vi "PIDByError.vi"(0 "Error":dbl, 1 "PID Gains":cluster{"P":dbl, "I":dbl, "D":dbl}, 2 "Init":bool, 3 "Reset":bool) -> (7 "Control":dbl)   [LabVIEW 2013, in "ProcessorHelperFunctions.lvlib"]
uses:
  ProcessorHelperFunctions.lvlib
  <vilib>/ptbypt/NI_PtbyPt.lvlib
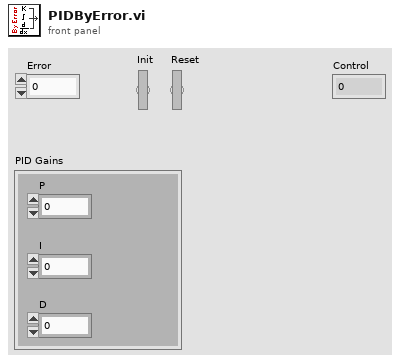
[diagram p1: front panel]
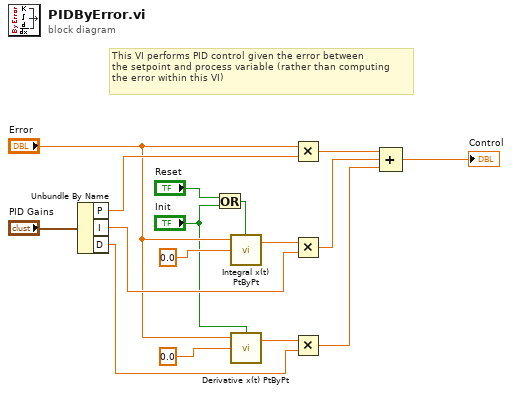
[diagram p0: block diagram]
diagram:
  # "This VI performs PID control given the error between\nthe setpoint and process variable (rather than computing\nthe error within this VI)"
  n1 = Unbundle By Name("PID Gains") -> ("P"=w15:dbl, "I"=w11:dbl, "D"=w7:dbl)
  n2 = Or(x="Reset", y="Init") -> (x .or. y?=w2:bool)
  n3 = call <vilib>:"Integral x(t) PtByPt.vi"("initialize"=w2, "initial condition"=0.0, "x"="Error") -> ("integral x(t)"=w10:dbl)  [unwired: 1 in, 1 out]
  n4 = call <vilib>:"Derivative x(t) PtByPt.vi"("initialize"="Init", "initial condition"=0.0, "x"="Error") -> ("dx/dt"=w6:dbl)  [unwired: 1 in, 1 out]
  n5 = Multiply(x="Error", y=w15) -> (x*y=w13:dbl)
  n6 = Multiply(x=w10, y=w11) -> (x*y=w9:dbl)
  n7 = Multiply(x=w6, y=w7) -> (x*y=w5:dbl)
  n8 = Compound Arithmetic op=ADD(w13, w9, w5) -> (→"Control":dbl)
